vi "Get Size (multiple).vi"(8 "error in (no error)":errorcluster, 11 "XY-data":cluster{"X-array":dbl[], "Y-array":dbl[]}[](array[cluster])) -> (0 "error out":errorcluster, 1 "X size":i32[](array[numeric]), 2 "Y size":i32[](array[numeric]), 3 "XY-data out":cluster{"X-array":dbl[], "Y-array":dbl[]}[](array[cluster]))   [LabVIEW 2019, in "xy_utilities.lvlib"]
uses:
  xy_utilities.lvlib
  Get X and Y.vi
  Get X and Y (single).vi
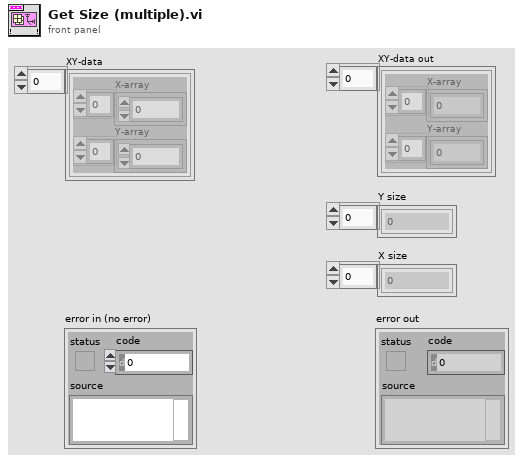
[diagram p1: front panel]
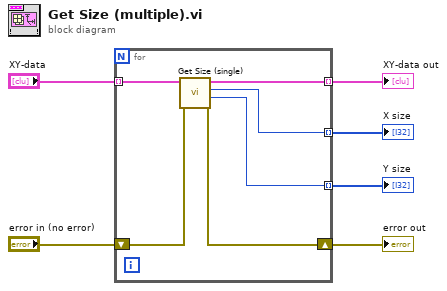
[diagram p0: block diagram]
diagram:
  n1 = for {
    tunnel: "XY-data" -> [w12] mode=indexing
    tunnel: [w11] -> w5 mode=indexing
    tunnel: [w10] -> w4 mode=indexing
    tunnel: [w9] -> w3 mode=indexing
    shift-right: [w8] -> w2
    shift-left: "error in (no error)" -> [w7]
    n2 = call "Get Size (single).vi"("error in (no error)"=w7, "XY-data"=w12) -> ("error out"=w8:errorcluster, "X size"=w9:i32, "Y size"=w10:i32, "XY-data out"=w11:cluster{"X-array":dbl[], "Y-array":dbl[]})  [unwired: 6 in]
  }
  "Y size" <- w3
  "X size" <- w4
  "error out" <- w2
  "XY-data out" <- w5
